vi "CRYReplace Analysis Curve Name.vi"(7 "Setup in":T1={"No.VI"=0, "Category"="", "StepName"="", "Seq setup flattened"="", "Comment"="", "Steps config."=[], "Jump config"=[], "Start"=0.0, "Increment"=0.0, "Name"="Pa", "Unit"="Pa", "Y data"=1, "Y prefix"="", "Y dB ref"=1.0, "Y unit"="", "Repeat State Array"=[]} {"Repeat State Array"."Start" format="%#_5g"; "Y dB ref" format="%.1f"; "Y data" items=["dB", "Lin"]; "Start" format="%#_5g"}, 8 "Hardware Setup In":string, 9 "Step Setup In":string, 10 "InsertSocket?":bool, 11 "Type In":string) -> (0 "New Custom Name( Channel case)":string[](array[string]), 1 "Signal Type":string, 2 "Curve Info Array Out":T2(array[cluster]), 3 "Inserted Names Out":string[](array[string]), 5 "New Custom Type( Channel case)":string[](array[string]))   [LabVIEW 2013]
uses:
  Typedef Control/CRYData Cluster Array.ctl
  Typedef Control/CRYData Cluster.ctl
  Typedef Control/CRYWaveform Cluster.ctl
  Typedef Control/CRYStep.ctl
  Typedef Control/CRYAnalysis CurveName Cluster.ctl
  Typedef Control/CRYUnit Info Out Cluster.ctl
panel:
  in  "Wave out":T3[](array[typedef]) {"Y dB ref" format="%.1f"; "Y axis" items=["Log", "Lin"]; "Y data" items=["dB", "Lin"]; "X data" items=["dB", "Lin"]}
  in  "Curve array":T4 {"Z data" items=["dB", "Lin"]; "X data" items=["dB", "Lin"]; "Y data" items=["dB", "Lin"]; "Z dB ref" format="%.1f"; "Z axis" items=["Log", "Lin"]; "X dB ref" format="%.1f"; "X axis" items=["Log", "Lin"]; "Y axis" items=["Log", "Lin"]; "Y dB ref" format="%.1f"; "Curve"."z" format="%.2f"; "Curve"."y" format="%.2f"; "Curve"."x" format="%.2f"}
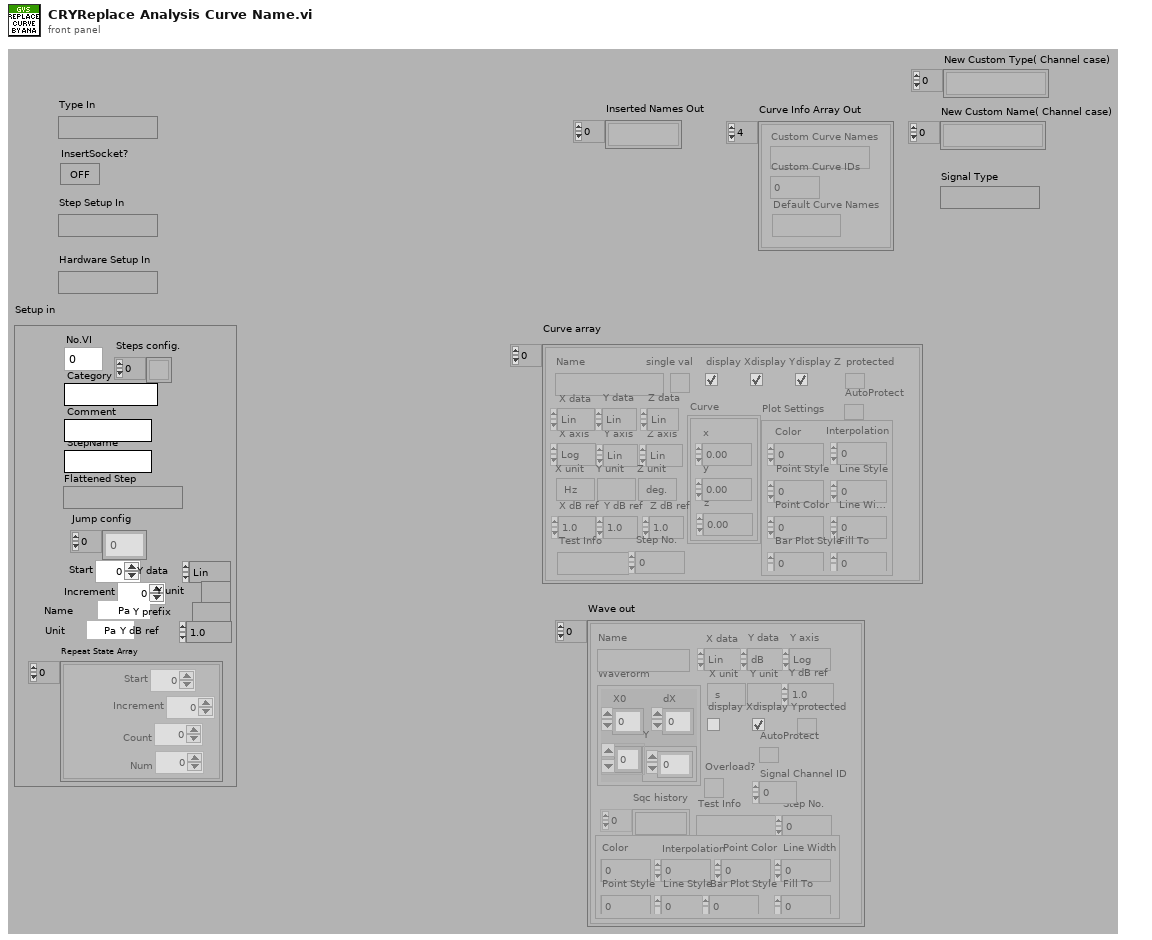
[diagram p1: front panel]
types:
  T1 = typedef "CRYStep.ctl" = cluster{"No.VI":i32, "Category":string, "StepName":string, "Seq setup flattened":string, "Comment":string, "Steps config.":bool[], "Jump config":i32[], "Start":dbl, "Increment":dbl, "Name":string, "Unit":string, "Y data":u16, "Y prefix":string, "Y dB ref":dbl, "Y unit":string, "Repeat State Array":cluster{"Start":dbl, "Increment":dbl, "Count":i32, "Num":i32}[]}
  T2 = cluster{"Custom Curve Names":string, "Custom Curve IDs":i32, "Default Curve Names":string}[]
  T3 = typedef "CRYWaveform Cluster.ctl" = cluster{"Waveform":cluster{"X0":dbl, "dX":dbl, "Y":sgl[]}, "X data":u16, "Y data":u16, "Y axis":u16, "X unit":string, "Y unit":string, "Y dB ref":dbl, "display Y":bool, "display X":bool, "Overload?":bool, "Test Info":string, "Step No.":i32, "Name":string, "protected":bool, "Sqc history":string[], "Signal Channel ID":i32, "Plot Settings":cluster{"Color":u32, "Interpolation":u8, "Point Style":u8, "Line Style":u8, "Point Color":u32, "Line Width":u8, "Bar Plot Style":u8, "Fill To":i16}, "AutoProtect":bool}
  T4 = typedef "CRYData Cluster Array.ctl" = T5[]
  T5 = typedef "CRYData Cluster.ctl" = cluster{"Name":string, "Curve":cluster{"x":dbl, "y":dbl, "z":dbl}[], "X data":u16, "Y data":u16, "Z data":u16, "X axis":u16, "Y axis":u16, "Z axis":u16, "X unit":string, "Y unit":string, "Z unit":string, "X dB ref":dbl, "Y dB ref":dbl, "Z dB ref":dbl, "single val":bool, "protected":bool, "display X":bool, "display Y":bool, "display Z":bool, "Test Info":string, "Step No.":i32, "Plot Settings":cluster{"Color":u32, "Interpolation":u8, "Point Style":u8, "Line Style":u8, "Point Color":u32, "Line Width":u8, "Bar Plot Style":u8, "Fill To":i16}, "AutoProtect":bool}
  T6 = cluster{"X unit":string, "X data":u16, "Y unit":string, "Y data":u16, "Z unit":string, "X data":u16, "dB ref":dbl}
  T7 = typedef "CRYUnit Info Out Cluster.ctl" = cluster{"X unit":string, "X data":u16, "Y unit":string, "Y data Time":u16, "Z unit":string, "X axis":u16, "X dB ref":dbl, "Y dB ref":dbl, "single/curve":bool}
  T8 = typedef "CRYAnalysis CurveName Cluster.ctl" = cluster{"Custom Curve Name":string, "Custom Curve ID":i32, "Default Curve Name":string}[]
  T9 = cluster{"display X":bool, "display Y":bool, "display Z":bool}[]
  T10 = cluster{"X unit":string, "X data":u16, "Y unit":string, "Y data":u16, "Z unit":string, "X data":u16, "dB ref":dbl}[]
  T11 = cluster{"Start":dbl, "Increment":dbl, "Count":i32, "Num":i32}[]
  T12 = typedef "CRYAnalysis Cluster.ctl" = cluster{"Name":string, "Harmonics":dbl[], " Algorithm":u16, "delay":dbl, "THD(%)":bool, "Rub&Buzz":bool, "Imp":bool, "Imp Ref resistor":dbl, "Y data":u16, "Y prefix":string, "Y unit":string, "Y dB ref":dbl, "Custom Curve Names":string[], "har list items":string[], "Envelope":bool, "use custom unit":bool, "autodelay ch":dbl, "impulse":bool, " start ms":dbl, " stop ms":dbl, "Scaling":i32, "Default Overlap ":bool, "Advanced View":bool, "Loose Particle":bool, "Use default":bool, "Auto-Correlation(Stimulus)":bool, "Auto-Correlation(Response)":bool, "Deconvolved Response":bool, "Mic Current":bool, "M List Vaiues":u16, "Type":u16, "Delay Method":u16, "Apply Correction Out":bool, "Apply Correction In":bool, "Harmonics @ meas.frq":bool, "THD Normalized(%)":bool, "Total Distortion":bool, "THD+Noise(%)":bool, "Rub&Buzz Norm'd(%)":bool, "Standard Error":bool, "Confidence Limits":bool, "Total Diff":bool, "Total Noise":bool, "Total DFD(%)":bool, "Total IMD(%)":bool, "Total IM":bool, "Total DFD+Noise(%)":bool, "Use Channel Name":bool, "Waveform In":string, "Waveform Out":string, "Method":u16, "Spectral Scaling":u16, "Appliied Unit":u16, "Length Unit":u16, "Applied Units":u16, "Sens Item":u16, "Tab":i32, "Distance Unit":u16, "discard cycles":dbl, "Weigting":string, "Averaging Time":dbl, "Max duration":dbl, "Min duration":dbl, "Attack Threshold":dbl, "Hysteresis Up":dbl, "Fmin(Hz)":dbl, "Fmax(Hz)":dbl, "Freq.Resolution":dbl, "Over-samples Res.":dbl, "Win Resolution":dbl, "distance":dbl, "samples":dbl, "Overlap":dbl, "Record Length":dbl, "No.of FFTs":dbl, "Hz":dbl, "record delay":dbl, " Std Err":dbl, "Response":bool, "Coherent Power*":bool, "Stimulus":bool, "Measurement Confidence":bool, "Auto Spectrum(Response)*":bool, "Auto Spectrum(Stimulus)*":bool, "Cross Spectrum*":bool, "functions":bool, "Frequency Response":bool, "Non-Coherent Power*":bool, "Coherence (%)":bool, "Non-Coherence (%)":bool, "Signal-Noise Ratio (dB)":bool, "Non-Coherenct Distirtion*":bool, "Result Waveforms":bool, "Coupling":bool, "Averaging":u16, "Harmonics":i32, "Custom Curve Names":i32, "unLabel":string, "Custom Curve Names":string, "Unit":string, "Total IMD + Noise(%) ":bool, "ResponseMe":u16, "Intermod":dbl[], "Diff\n":dbl[], "Cross-Correlation":bool, "IM list items":string[], "Diff list items":string[], "TSR Window Type":string, "Help":string, "Custom Curve IDs":i32[], "Default Curve Names":string[], "Loose Particle waveform":bool, "Perceptual Rub&Buzz":bool, "Imp Auto Mode":u16, "Mic Auto Mode":u16, "Mic Ref resistor":dbl, "Curve Resolution":u16, "Curve Resolution Hz":dbl, "Polarity":bool}
  T13 = typedef "CRYStimulus Test Infor Cluster.ctl" = cluster{"Stimulus Type":string, "Signal Type":string, "In/Out":bool, "FAPS":cluster{"freq":dbl, "ampl":dbl, "cycles":dbl, "samples":i32}[], "Sampling Rate":dbl, "Samples":i32, "Analysis Param":string, "Resolution":u16, "Steps":u32, "Analysis Value":dbl[], "Diff Freq":dbl, "FStart":dbl, "FStop":dbl, "Calibration Param":string, "Anti Alias":dbl, "Level Out1":dbl, "Level Out2":dbl, "EQ":bool}
  T14 = typedef "CRYCalibration 2DCluster.ctl" = cluster{"Calibration":T15, "Corr Curve":T5, "EQ Curve":T5, "Sens Curve":T5}
  T15 = typedef "CRYCalibration Cluster.ctl" = cluster{"Calibration Step Name":string, "Device":string, "Correction Curve Name":string, "Equalization Curve Name":string, "Sensitivity Curve Name":string, "Corr Folder and File":string, "EQ Folder and File":string, "Sens Folder and File":string, "Corr Step size":u16, "EQ Step size":u16, "Input":bool, "Last Cal Date (sec)":timestamp, "Cha Name":string, "Corr Curve Found":bool, "EQ Curve Found":bool, "Sens Curve Found":bool, "Signal Type":string, "Calibrated Device":string, "Hz":u32}
  T16 = cluster{bool, "Check Option":string, "use custom unit":bool, "Custom Curve Names":string[], "Custom Curve IDs":i32[], "Default Curve Names":string[], "Use default":bool}
  T17 = cluster{"Y unit":string, "Y dB ref":dbl, "Y unit":string, "Y dB ref":dbl, "Y unit":string, "Y dB ref":dbl, "Y data":u16, u16}
  T18 = cluster{"X unit":string, "X data":u16, "Y unit":string, "X data":u16, "Y unit":string, "X data":u16, "dB ref In":dbl}[]
  T19 = cluster{"X unit":string, "X data":u16, "Y unit":string, "Y data Time":u16, "Z unit":string, "X data":u16, "dB ref":dbl}[]
  T20 = typedef "CRYWaveform Cluster Array.ctl" = T3[]
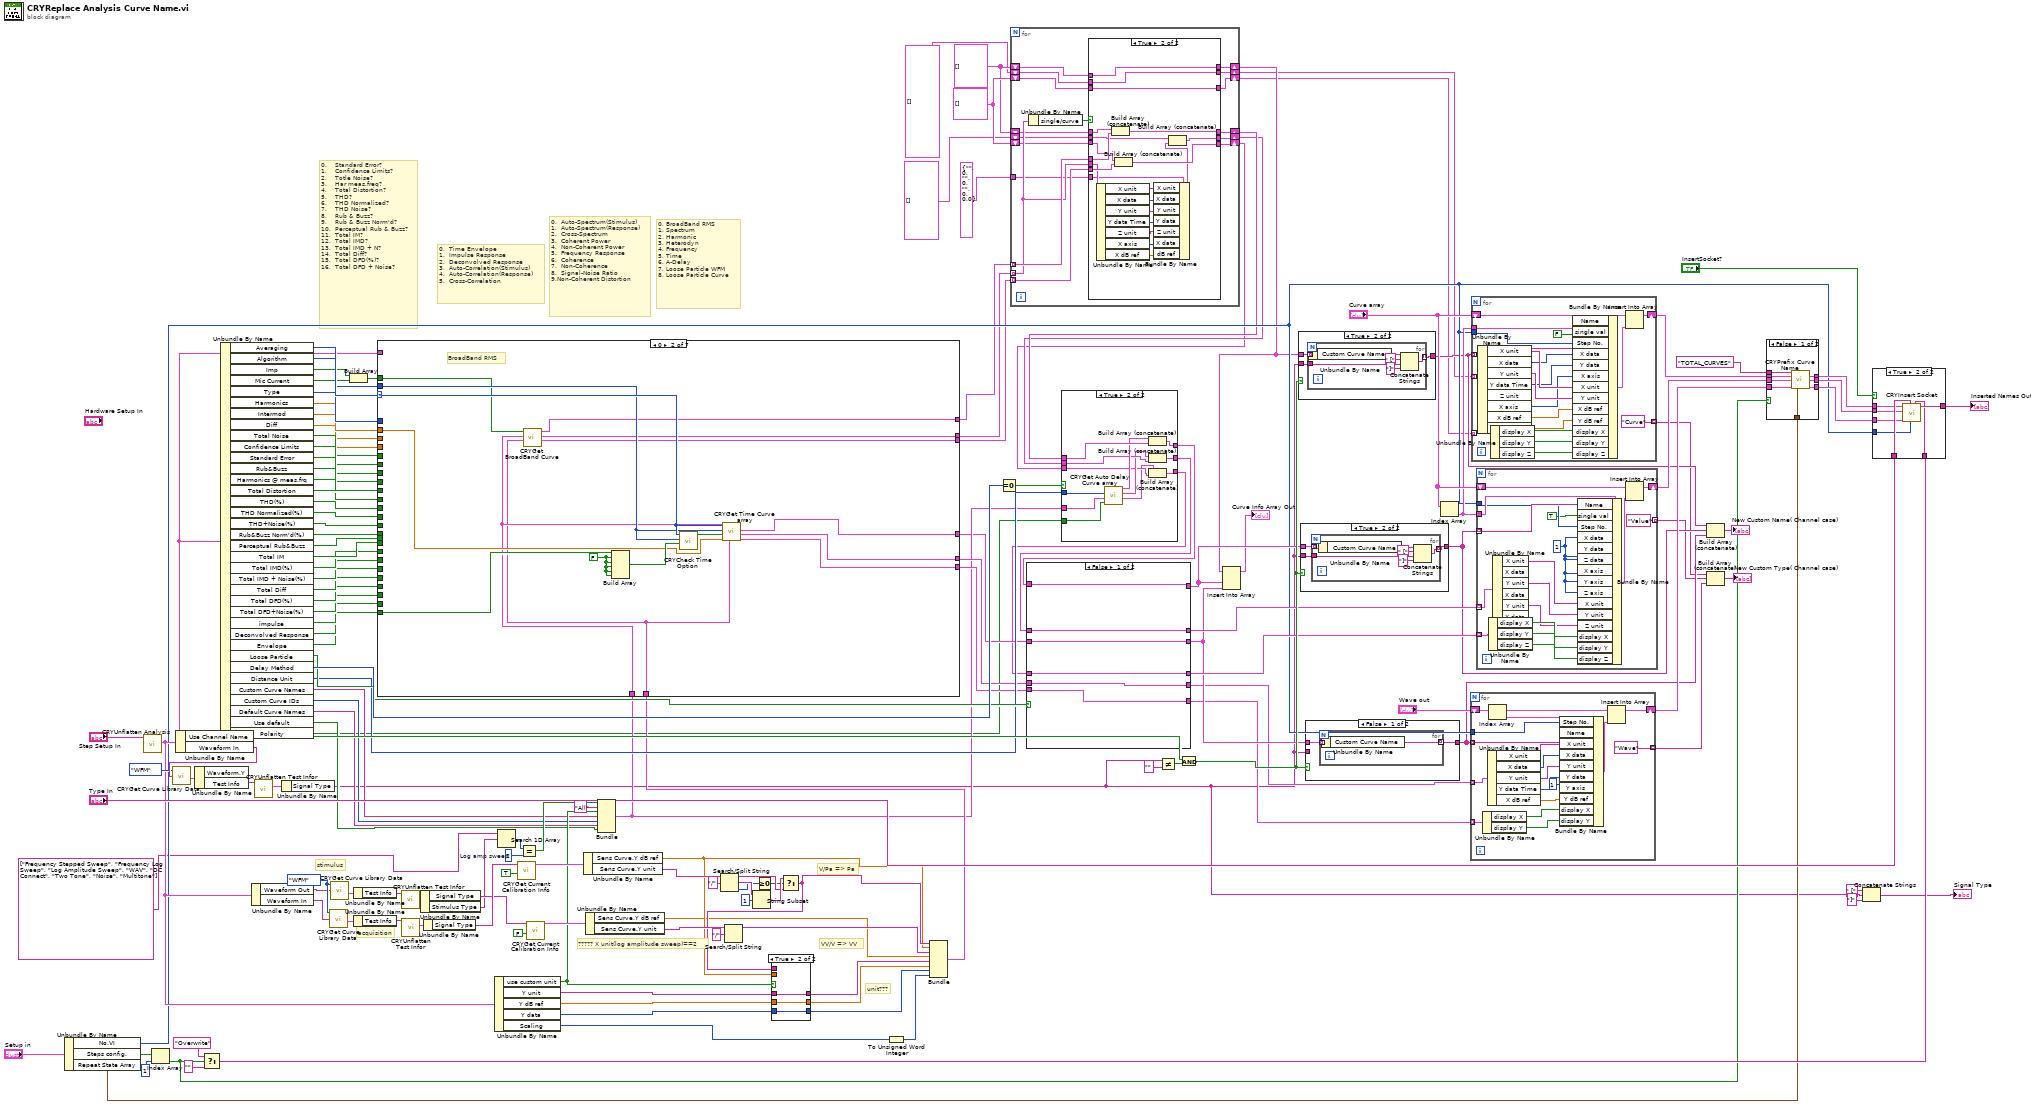
[diagram p0: block diagram]
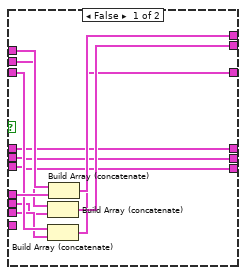
[diagram p2: hidden frame]
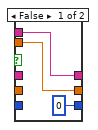
[diagram p5: hidden frame]
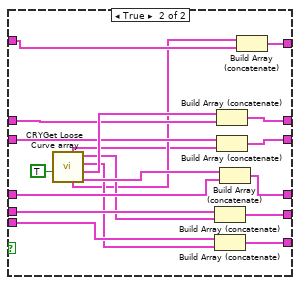
[diagram p7: hidden frame]
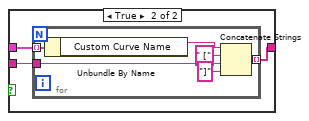
[diagram p8: hidden frame]
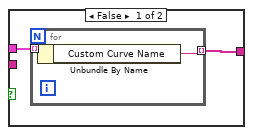
[diagram p9: hidden frame]
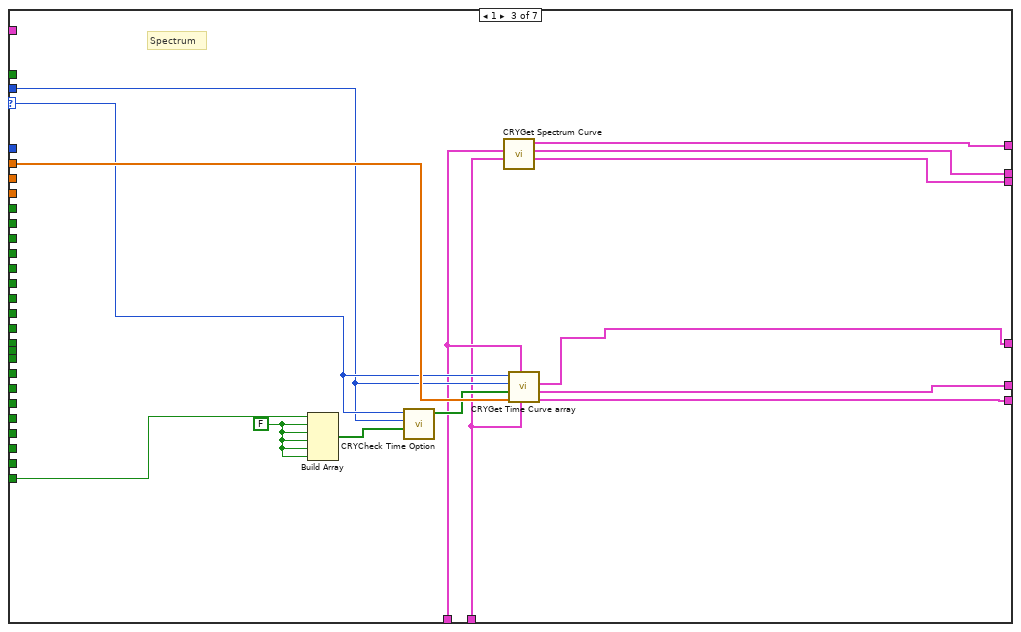
[diagram p11: hidden frame]
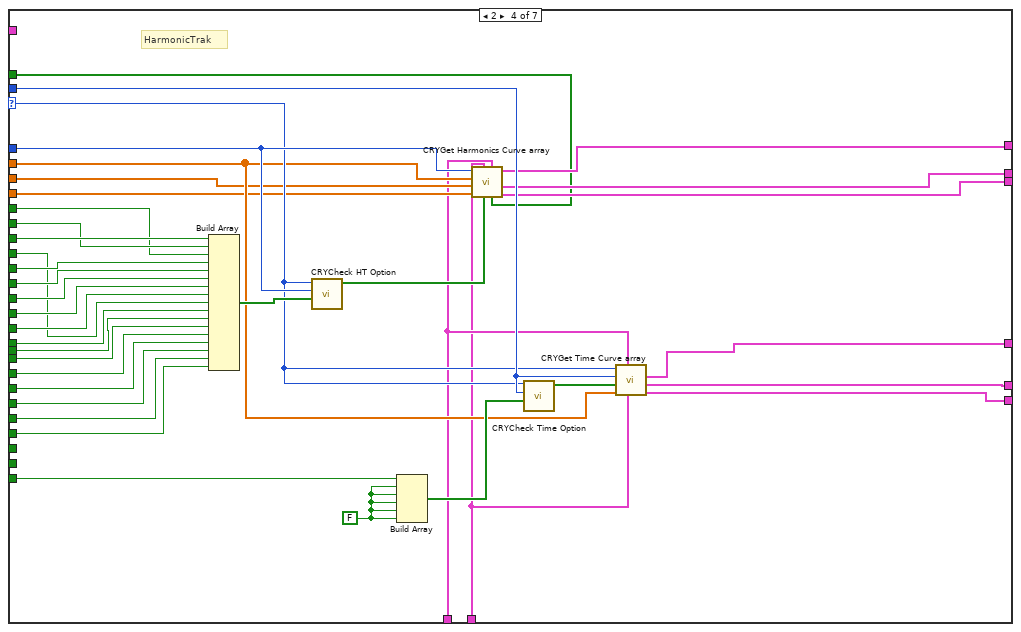
[diagram p12: hidden frame]
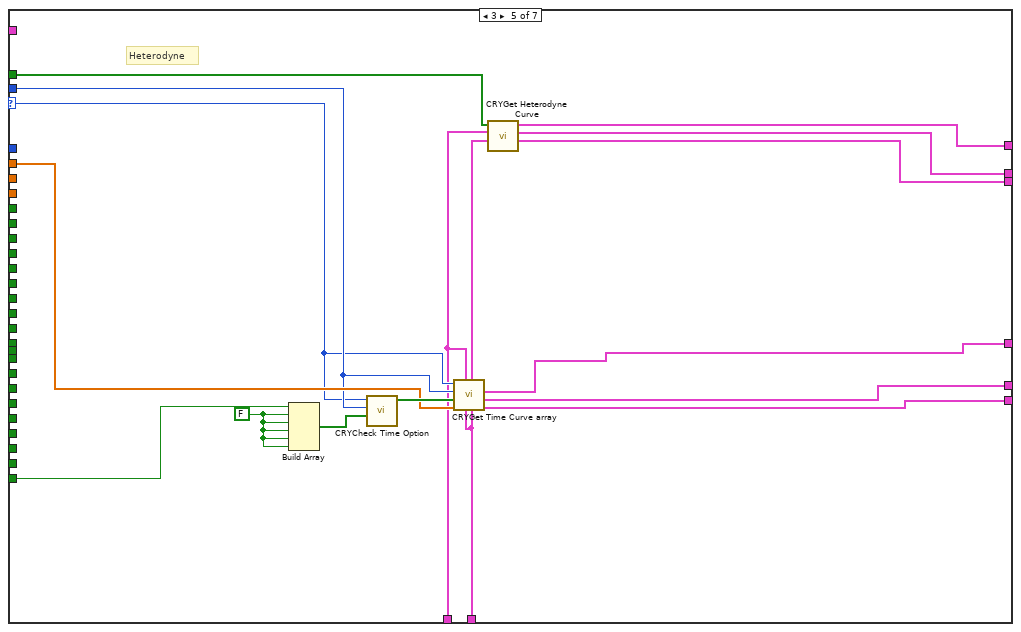
[diagram p13: hidden frame]
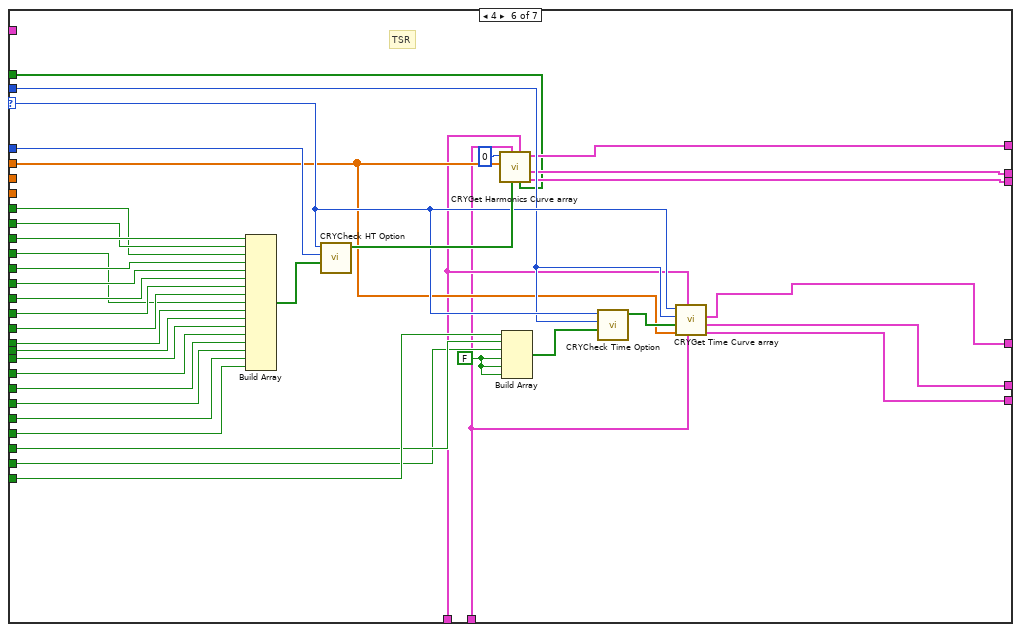
[diagram p14: hidden frame]
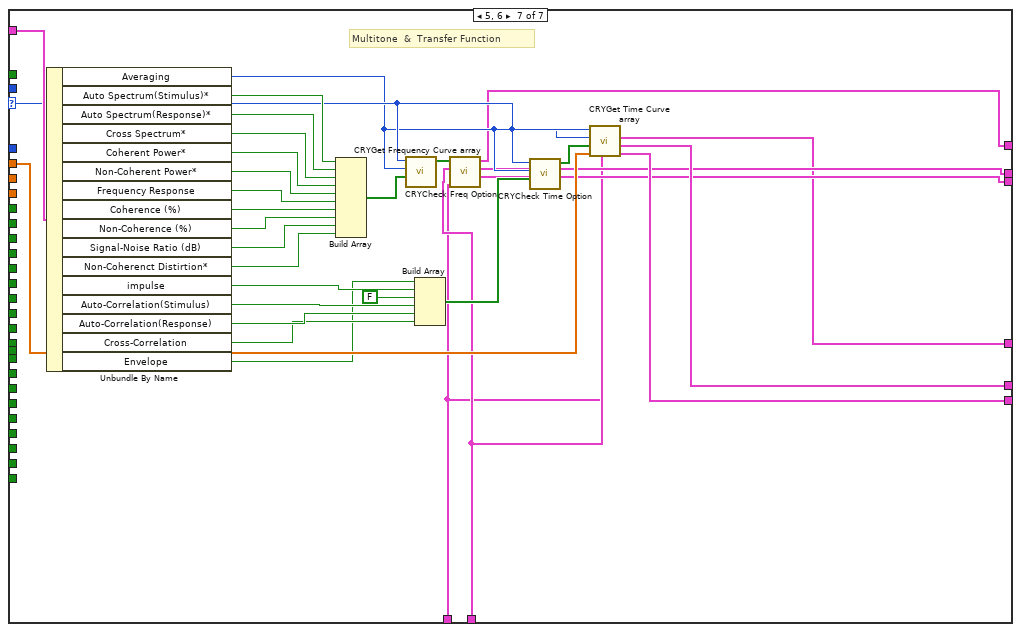
[diagram p15: hidden frame]
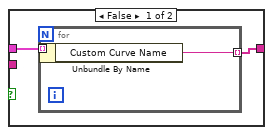
[diagram p16: hidden frame]
diagram:
  w13 = T8 [] ("Curve Info Array Out")
  w15 = T9 []
  w72 = 2  # Log amp sweep
  w82 = enum16{"Curves", "Values", "Results", "WFM"}."WFM" ("Type")
  # "0, BroadBand RMS\n1, Spectrum\n2, Harmonic\n3, Heterodyn\n4, Frequency\n5, Time\n6, A-Delay\n7, Loose Particle WFM\n8, Loose Particle Curve"
  # "acquisition"
  # "stimulus"
  # "unit???"
  # "V/Pa => Pa"
  # "VV/V => VV"
  # "????? X unit(log amplitude sweep)==2"
  # "0,  Auto-Spectrum(Stimulus)\n1,  Auto-Spectrum(Response)\n2,  Cross-Spectrum\n3,  Coherent Power\n4,  Non-Coherent Power\n5,  Frequency Response\n6,  Coherence\n7,  Non-Coherence\n8,  Signal-Noise Ratio\n9,Non-Coherent Distortion"
  # "0,    Standard Error?\n1,    Confidence Limits?\n2,    Totle Noise?\n3,    Har meas.freq?\n4,    Total Distortion?\n5,    THD?\n6,    THD Normalized?\n7,    THD Noise?\n8,    Rub & Buzz?\n9,    Rub & Buzz Norm'd?\n10,  Perceptual Rub & Buzz?\n11,  Total IM?\n12,  Total IMD?\n13,  Total IMD + N?\n14,  Total Diff?\n15,  Total DFD(%)?\n16,  Total DFD + Noise?"
  # "0,  Time Envelope\n1,  Impulse Response\n2,  Deconvolved Response\n3,  Auto-Correlation(Stimulus)\n4,  Auto-Correlation(Response)\n5,  Cross-Correlation"
  n1 = Unbundle By Name("Setup in") -> ("No.VI"=w37:i32, "Steps config."=w47:bool[], "Repeat State Array"=w39:T11)
  n2 = call "CRYUnflatten Analysis.vi"("Unflatten Analysis"="Step Setup In") -> ("Analysis"=w75:T12)  [unwired: 8 in, 2 out]
  n3 = Index Array(array=w47, index=1) -> (element=w38:bool)
  n4 = Unbundle By Name(w75) -> ("Use Channel Name"=w124:bool, "Waveform In"=w155:string)
  n5 = call "CRYGet Curve Library Data.vi"("Type"=enum16{"Curves", "Values", "Results", "WFM"}."WFM", "Data Name"=w155) -> ("Wave"=w153:T3)  [unwired: 4 out]
  n6 = Unbundle By Name(w153) -> ("Test Info"=w152:string)  [unwired: 1 out]
  n7 = Select(t="Overwrite" ("Y unit"), s=w38, f="") -> (s? t:f=w49:string)
  n8 = Unbundle By Name(w75) -> ("Averaging"=w120:u16, "Algorithm"=w150:u16, "Imp"=w22:bool, "Mic Current"=w21:bool, "Type"=w149:u16, "Harmonics"=w148:dbl[], "Intermod"=w137:dbl[], "Diff"=w133:dbl[], "Total Noise"=w138:bool, "Confidence Limits"=w139:bool, "Standard Error"=w140:bool, "Rub&Buzz"=w141:bool, "Harmonics @ meas.frq"=w147:bool, "Total Distortion"=w146:bool, "THD(%)"=w145:bool, "THD Normalized(%)"=w144:bool, "THD+Noise(%)"=w143:bool, "Rub&Buzz Norm'd(%)"=w142:bool, "Perceptual Rub&Buzz"=w35:bool, "Total IM"=w136:bool, "Total IMD(%)"=w135:bool, "Total IMD + Noise(%)"=w134:bool, "Total Diff"=w132:bool, "Total DFD(%)"=w131:bool, "Total DFD+Noise(%)"=w130:bool, "impulse"=w129:bool, "Deconvolved Response"=w128:bool, "Envelope"=w121:bool, "Loose Particle"=w116:bool, "Delay Method"=w127:u16, "Distance Unit"=w114:u16, "Custom Curve Names"=w60:string[], "Custom Curve IDs"=w59:i32[], "Default Curve Names"=w58:string[], "Use default"=w57:bool, "Polarity"=w19:bool)
  n9 = Unbundle By Name(w75) -> ("Waveform Out"=w80:string, "Waveform In"=w81:string)
  n10 = call "CRYUnflatten Test Infor.vi"("Falattend test infor"=w152) -> ("unflattened test infor data"=w151:T13)  [unwired: 9 out]
  n11 = Unbundle By Name(w151) -> ("Signal Type"=w28:string)
  n12 = call "CRYGet Curve Library Data.vi"("Type"=w82, "Data Name"=w81) -> ("Wave"=w84:T3)  [unwired: 4 out]
  n13 = call "CRYGet Curve Library Data.vi"("Type"=w82, "Data Name"=w80) -> ("Wave"=w83:T3)  [unwired: 4 out]
  n14 = Build Array(w22, w21) -> (w20:bool[])
  n15 = Unbundle By Name(w83) -> ("Test Info"=w76:string)
  n16 = Unbundle By Name(w84) -> ("Test Info"=w78:string)
  n17 = call "CRYUnflatten Test Infor.vi"("Falattend test infor"=w76) -> ("unflattened test infor data"=w79:T13)  [unwired: 9 out]
  n18 = call "CRYUnflatten Test Infor.vi"("Falattend test infor"=w78) -> ("unflattened test infor data"=w77:T13)  [unwired: 9 out]
  n19 = Unbundle By Name(w79) -> ("Signal Type"=w73:string, "Stimulus Type"=w70:string)
  n20 = Unbundle By Name(w77) -> ("Signal Type"=w74:string)
  n21 = Unbundle By Name(w75) -> ("use custom unit"=w61:bool, "Y unit"=w95:string, "Y dB ref"=w96:dbl, "Y data"=w94:u16, "Scaling"=w93:i32)
  n22 = Search 1D Array(1D array=string[] ["Frequency Stepped Sweep", "Frequency Log Sweep", "Log Amplitude Sweep", "WAV", "DC Connect", "Two Tone", "Noise", "Multitone"] ("Strings []"), element=w70) -> (index of element=w71:i32)  [unwired: 1 out]
  n23 = call "CRYGet Current Calibration Info.vi"("Is Input?"=TRUE, "Signal Type Name"=w74) -> ("Calibration All Cluster"=w106:T14)  [unwired: 9 out]
  n24 = Equal?(x=w71, y=w72) -> (x = y?=w69:bool)
  n25 = call "CRYGet Current Calibration Info.vi"("Is Input?"=FALSE, "Signal Type Name"=w73) -> ("Calibration All Cluster"=w109:T14)  [unwired: 9 out]
  n26 = Unbundle By Name(w106) -> ("Sens Curve.Y dB ref"=w90:dbl, "Sens Curve.Y unit"=w97:string)
  n27 = Unbundle By Name(w109) -> ("Sens Curve.Y dB ref"=w88:dbl, "Sens Curve.Y unit"=w105:string)
  n28 = Bundle(w69, "Check Option"="All", "use custom unit"=w61, "Custom Curve Names"=w60, "Custom Curve IDs"=w59, "Default Curve Names"=w58, "Use default"=w57) -> (w56:T16)  [unwired: 1 in]
  n29 = Search/Split String(string=w97, search string/char (-)="/" ("search char (-)")) -> (substring before match=w101:string, match + rest of string=w103:string, offset of match=w99:i32)  [unwired: 1 out]
  n30 = Search/Split String(string=w105, search string/char (-)="/" ("search char (-)")) -> (substring before match=w89:string)  [unwired: 3 out]
  n31 = String Subset(string=w103, offset (0)=1) -> (substring=w104:string)  [unwired: 1 in]
  n32 = Greater Or Equal To 0?(x=w99) -> (x >= 0?=w100:bool)
  n33 = Select(t=w104, s=w100, f=w101) -> (s? t:f=w91:string)
  n34 = case shown="True" w61 {
    tunnel: w96 -> [_ w161]
    tunnel: w95 -> [_ w162]
    tunnel: [w158 w162] -> w87
    tunnel: w90 -> [w159 _]
    tunnel: w91 -> [w158 _]
    tunnel: [w159 w161] -> w86
    tunnel: w94 -> [_ w160]
    tunnel: [u16 0 ("Y data") w160] -> w85
    frame False {
    }
    frame True {
    }
  }
  n35 = To Unsigned Word Integer(number=w93) -> (unsigned 16bit integer=w92:u16)
  n36 = Bundle("Y unit"=w91, "Y dB ref"=w90, "Y unit"=w89, "Y dB ref"=w88, "Y unit"=w87, "Y dB ref"=w86, "Y data"=w85, w92) -> (w67:T17)  [unwired: 1 in]
  n37 = case shown="0" w150 {
    selector: w150 -> [_ w173 w188 w207 w241 w260 w299]
    tunnel: w149 -> [_ _ _ w214 _ w268 _]
    tunnel: w148 -> [_ w174 w190 w206 w243 w258 w296]
    tunnel: w147 -> [_ _ _ w231 _ w282 _]
    tunnel: w146 -> [_ _ _ w230 _ w281 _]
    tunnel: w145 -> [_ _ _ w229 _ w280 _]
    tunnel: w144 -> [_ _ _ w228 _ w279 _]
    tunnel: w143 -> [_ _ _ w227 _ w278 _]
    tunnel: w142 -> [_ _ _ w226 _ w276 _]
    tunnel: w141 -> [_ _ _ w225 _ w277 _]
    tunnel: w140 -> [_ _ _ w224 _ w285 _]
    tunnel: w139 -> [_ _ _ w223 _ w284 _]
    tunnel: w138 -> [_ _ _ w216 _ w283 _]
    tunnel: w137 -> [_ _ _ w205 _ _ _]
    tunnel: w136 -> [_ _ _ w222 _ w275 _]
    tunnel: w135 -> [_ _ _ w221 _ w274 _]
    tunnel: w134 -> [_ _ _ w220 _ w273 _]
    tunnel: w133 -> [_ _ _ w204 _ _ _]
    tunnel: w132 -> [_ _ _ w219 _ w272 _]
    tunnel: w131 -> [_ _ _ w218 _ w271 _]
    tunnel: w130 -> [_ _ _ w217 _ w270 _]
    tunnel: w129 -> [_ _ _ _ _ w265 _]
    tunnel: w128 -> [_ _ _ _ _ w264 _]
    tunnel: w75 -> [_ _ _ _ _ _ w318]
    tunnel: [_ w166 w181 w198 w235 w252 w288] -> w18
    tunnel: [_ w167 w182 w199 w236 w253 w289] -> w55
    tunnel: w121 -> [_ w177 w192 w211 w247 w266 _]
    tunnel: w120 -> [_ w172 w187 w208 w242 w259 _]
    tunnel: w56 -> [_ w165 w180 w197 w234 w251 w287]
    tunnel: w67 -> [_ w164 w179 w196 w233 w250 w290]
    tunnel: [_ w171 w186 w201 w238 w255 w294] -> w65
    tunnel: [_ w170 w185 w200 w237 w254 w293] -> w64
    tunnel: [_ w169 w184 w203 w240 w257 w291] -> w17
    tunnel: [_ w168 w183 w202 w239 w256 w292] -> w16
    tunnel: w35 -> [_ _ _ w195 _ w249 _]
    tunnel: w20 -> [_ w163 _ w194 w232 w248 _]
    frame Default {
    }
    frame 0 {
      w178 = FALSE ("element")
      # "BroadBand RMS"
      n38 = call "CRYGet BroadBand Curve.vi"("Unit Info In"=w164, "Additive Info"=w165, "Impedance and Mic Current In"=w163) -> ("Display Array"=w168:T9, "Unit Info Out"=w169:T7[], "Curve Info Array Out"=w166:T8)  [unwired: 6 in]
      n39 = Build Array(w177, w178, w178, w178, w178, w178) -> (w176:bool[])
      n40 = call "CRYCheck Time Option.vi"("Option Array In"=w176, "Averaging"=w172, "Algorithm"=w173) -> ("Option Array Out"=w175:bool[])  [unwired: 8 in]
      n41 = call "CRYGet Time Curve array.vi"("Unit Info In"=w164, "Additive Info"=w165, "Harmonics array"=w174, "Option Array In"=w175, "Averaging"=w172, "Algorithm"=w173) -> ("Display Array"=w170:T9, "Unit Info Out"=w171:T7[], "Curve Info Array Out"=w167:T8)  [unwired: 3 in]
    }
    frame 1 {
      w193 = FALSE ("element")
      # "Spectrum"
      n42 = Build Array(w192, w193, w193, w193, w193, w193) -> (w191:bool[])
      n43 = call "CRYCheck Time Option.vi"("Option Array In"=w191, "Averaging"=w187, "Algorithm"=w188) -> ("Option Array Out"=w189:bool[])  [unwired: 8 in]
      n44 = call "CRYGet Spectrum Curve.vi"("Unit Info In"=w179, "Additive Info"=w180) -> ("Display Array"=w183:T9, "Unit Info Out"=w184:T7[], "Curve Info Array Out"=w181:T8)  [unwired: 7 in]
      n45 = call "CRYGet Time Curve array.vi"("Unit Info In"=w179, "Additive Info"=w180, "Harmonics array"=w190, "Option Array In"=w189, "Averaging"=w187, "Algorithm"=w188) -> ("Display Array"=w185:T9, "Unit Info Out"=w186:T7[], "Curve Info Array Out"=w182:T8)  [unwired: 3 in]
    }
    frame 2 {
      w212 = FALSE ("element")
      # "HarmonicTrak"
      n46 = Build Array(w224, w223, w216, w231, w230, w229, w228, w227, w225, w226, w195, w222, w221, w220, w219, w218, w217) -> (w215:bool[])
      n47 = call "CRYCheck HT Option.vi"("Option Array In"=w215, "Type"=w214, "Algorithm"=w207) -> ("Option Array Out"=w213:bool[])  [unwired: 8 in]
      n48 = Build Array(w211, w212, w212, w212, w212, w212) -> (w210:bool[])
      n49 = call "CRYGet Harmonics Curve array.vi"("Impedance and Mic Current In"=w194, "Additive Info"=w197, "Option Array In"=w213, "Unit Info"=w196, "Diff array"=w204, "IM array"=w205, "Harmonics array"=w206, "Type"=w214) -> ("Display Array"=w202:T9, "Unit Info Out"=w203:T7[], "Curve Info Array Out"=w198:T8)  [unwired: 1 out]
      n50 = call "CRYCheck Time Option.vi"("Option Array In"=w210, "Averaging"=w208, "Algorithm"=w207) -> ("Option Array Out"=w209:bool[])  [unwired: 8 in]
      n51 = call "CRYGet Time Curve array.vi"("Unit Info In"=w196, "Additive Info"=w197, "Harmonics array"=w206, "Option Array In"=w209, "Averaging"=w208, "Algorithm"=w207) -> ("Display Array"=w200:T9, "Unit Info Out"=w201:T7[], "Curve Info Array Out"=w199:T8)  [unwired: 3 in]
    }
    frame 3 {
      w246 = FALSE ("element")
      # "Heterodyne"
      n52 = Build Array(w247, w246, w246, w246, w246, w246) -> (w245:bool[])
      n53 = call "CRYCheck Time Option.vi"("Option Array In"=w245, "Averaging"=w242, "Algorithm"=w241) -> ("Option Array Out"=w244:bool[])  [unwired: 8 in]
      n54 = call "CRYGet Time Curve array.vi"("Unit Info In"=w233, "Additive Info"=w234, "Harmonics array"=w243, "Option Array In"=w244, "Averaging"=w242, "Algorithm"=w241) -> ("Display Array"=w237:T9, "Unit Info Out"=w238:T7[], "Curve Info Array Out"=w236:T8)  [unwired: 3 in]
      n55 = call "CRYGet Heterodyne Curve.vi"("Unit Info In"=w233, "Additive Info"=w234, "Impedance and Mic Current In"=w232) -> ("Display Array"=w239:T9, "Unit Info Out"=w240:T7[], "Curve Info Array Out"=w235:T8)  [unwired: 6 in]
    }
    frame 4 {
      w263 = FALSE ("element")
      # "TSR"
      n56 = Build Array(w285, w284, w283, w282, w281, w280, w279, w278, w277, w276, w249, w275, w274, w273, w272, w271, w270) -> (w269:bool[])
      n57 = call "CRYCheck HT Option.vi"("Option Array In"=w269, "Type"=w268, "Algorithm"=w260) -> ("Option Array Out"=w267:bool[])  [unwired: 8 in]
      n58 = call "CRYGet Harmonics Curve array.vi"("Impedance and Mic Current In"=w248, "Additive Info"=w251, "Option Array In"=w267, "Unit Info"=w250, "Harmonics array"=w258, "Type"=u16 0) -> ("Display Array"=w256:T9, "Unit Info Out"=w257:T7[], "Curve Info Array Out"=w252:T8)  [unwired: 2 in, 1 out]
      n59 = Build Array(w266, w265, w264, w263, w263, w263) -> (w262:bool[])
      n60 = call "CRYCheck Time Option.vi"("Option Array In"=w262, "Averaging"=w259, "Algorithm"=w260) -> ("Option Array Out"=w261:bool[])  [unwired: 8 in]
      n61 = call "CRYGet Time Curve array.vi"("Unit Info In"=w250, "Additive Info"=w251, "Harmonics array"=w258, "Option Array In"=w261, "Averaging"=w259, "Algorithm"=w260) -> ("Display Array"=w254:T9, "Unit Info Out"=w255:T7[], "Curve Info Array Out"=w253:T8)  [unwired: 3 in]
    }
    frame 5, 6 {
      # "Multitone  &  Transfer Function"
      n62 = Unbundle By Name(w318) -> ("Averaging"=w298:u16, "Auto Spectrum(Stimulus)*"=w317:bool, "Auto Spectrum(Response)*"=w316:bool, "Cross Spectrum*"=w315:bool, "Coherent Power*"=w314:bool, "Non-Coherent Power*"=w313:bool, "Frequency Response"=w312:bool, "Coherence (%)"=w311:bool, "Non-Coherence (%)"=w310:bool, "Signal-Noise Ratio (dB)"=w309:bool, "Non-Coherenct Distirtion*"=w308:bool, "impulse"=w305:bool, "Auto-Correlation(Stimulus)"=w303:bool, "Auto-Correlation(Response)"=w302:bool, "Cross-Correlation"=w301:bool, "Envelope"=w295:bool)
      n63 = Build Array(w317, w316, w315, w314, w313, w312, w311, w310, w309, w308) -> (w307:bool[])
      n64 = call "CRYCheck Freq Option.vi"("Option Array In"=w307, "Averaging"=w298, "Algorithm"=w299) -> ("Option Array Out"=w306:bool[])  [unwired: 8 in]
      n65 = Build Array(w295, w305, FALSE ("element"), w303, w302, w301) -> (w300:bool[])
      n66 = call "CRYGet Frequency Curve array.vi"("Additive Info"=w287, "Unit Info In"=w290, "Option Array In"=w306) -> ("Display Array"=w292:T9, "Unit Info Out"=w291:T7[], "Curve Info Array Out"=w288:T8)  [unwired: 6 in]
      n67 = call "CRYCheck Time Option.vi"("Option Array In"=w300, "Averaging"=w298, "Algorithm"=w299) -> ("Option Array Out"=w297:bool[])  [unwired: 8 in]
      n68 = call "CRYGet Time Curve array.vi"("Unit Info In"=w290, "Additive Info"=w287, "Harmonics array"=w296, "Option Array In"=w297, "Averaging"=w298, "Algorithm"=w299) -> ("Display Array"=w293:T9, "Unit Info Out"=w294:T7[], "Curve Info Array Out"=w289:T8)  [unwired: 3 in]
    }
  }
  n69 = Equal To 0?(x=w127) -> (x = 0?=w115:bool)
  n70 = for {
    tunnel: w18 -> [w333] mode=indexing
    tunnel: w17 -> [w332] mode=indexing
    tunnel: w16 -> [w331] mode=indexing
    shift-right: [w325] -> w10
    shift-left: w13 -> [w334]
    shift-right: [w324] -> w9
    shift-left: T7[] [] -> [w327]
    shift-right: [w323] -> w8
    shift-left: w15 -> [w326]
    shift-right: [w322] -> w7
    shift-left: w13 -> [w330]
    shift-right: [w321] -> w6
    shift-left: T10 [] -> [w329]
    shift-right: [w320] -> w5
    shift-left: w15 -> [w328]
    tunnel: T6 {"X unit"="", "X data"=0, "Y unit"="", "Y data"=0, "Z unit"="", "X data"=0, "dB ref"=0.0} ("Value Unit Info Out") -> [w319]
    n71 = Unbundle By Name(w332) -> ("single/curve"=w335:bool)
    n72 = case shown="True" w335 {
      tunnel: w334 -> [w347 w368]
      tunnel: w333 -> [w346 w364]
      tunnel: w332 -> [w339 w357]
      tunnel: w331 -> [w340 w361]
      tunnel: w330 -> [w338 w365]
      tunnel: w329 -> [w337 w359]
      tunnel: w328 -> [w336 w362]
      tunnel: w327 -> [w344 w367]
      tunnel: w326 -> [w342 w366]
      tunnel: [w345 w368] -> w325
      tunnel: [w343 w367] -> w324
      tunnel: [w341 w366] -> w323
      tunnel: [w338 w363] -> w322
      tunnel: [w337 w358] -> w321
      tunnel: [w336 w360] -> w320
      tunnel: w319 -> [_ w348]
      frame False {
        n73 = Build Array (concatenate)(w344, w339) -> (w343:T7[])
        n74 = Build Array (concatenate)(w342, w340) -> (w341:T9)
        n75 = Build Array (concatenate)(w347, w346) -> (w345:T8)
      }
      frame True {
        n76 = Unbundle By Name(w357) -> ("X unit"=w356:string, "X data"=w355:u16, "Y unit"=w354:string, "Y data Time"=w353:u16, "Z unit"=w352:string, "X axis"=w351:u16, "X dB ref"=w350:dbl)
        n77 = Build Array (concatenate)(w365, w364) -> (w363:T8)
        n78 = Build Array (concatenate)(w362, w361) -> (w360:T9)
        n79 = Bundle By Name(cluster=w348, "X unit"=w356, "X data"=w355, "Y unit"=w354, "Y data"=w353, "Z unit"=w352, "X data"=w351, "dB ref"=w350) -> (w349:T6)
        n80 = Build Array (concatenate)(w359, w349) -> (w358:T10)
      }
    }
  }
  n81 = case shown="True" w115 {
    tunnel: w114 -> [_ w383]
    tunnel: w56 -> [_ w382]
    tunnel: w19 -> [_ w381]
    tunnel: w7 -> [w371 w380]
    tunnel: w6 -> [w370 w375]
    tunnel: w5 -> [w369 w373]
    tunnel: [w371 w379] -> w4
    tunnel: [w370 w378] -> w3
    tunnel: [w369 w377] -> w2
    frame False {
    }
    frame True {
      n82 = call "CRYGet Auto Delay Curve array.vi"("Polarity"=w381, "Additive Info"=w382, "Distance Unit"=w383) -> ("Value Display Array"=w372:T9, "Value Unit Info Out"=w374:T18, "Curve Info Array Out"=w376:T8)  [unwired: 6 in]
      n83 = Build Array (concatenate)(w376, w380) -> (w379:T8)
      n84 = Build Array (concatenate)(w374, w375) -> (w378:T10)
      n85 = Build Array (concatenate)(w372, w373) -> (w377:T9)
    }
  }
  n86 = case shown="False" w116 {
    tunnel: w55 -> [w385 w396]
    tunnel: [w385 w395] -> w66
    tunnel: w4 -> [w384 w393]
    tunnel: w3 -> [w389 w406]
    tunnel: w2 -> [w388 w404]
    tunnel: [w389 w394] -> w112
    tunnel: [w388 w408] -> w113
    tunnel: w65 -> [w387 w402]
    tunnel: w64 -> [w386 w400]
    tunnel: [w387 w398] -> w63
    tunnel: [w386 w397] -> w62
    tunnel: [w384 w392] -> w54
    frame False {
    }
    frame True {
      n87 = call "CRYGet Loose Curve array.vi"("Loose Particle Waveform"=TRUE) -> ("Value Display Array"=w405:T9, "Value Unit Info Out"=w407:T19, "WMF Display Array"=w399:T9, "WFM Unit Info Out"=w401:T7[], "Curve Info Array Out"=w391:T8, "WFM Info Array Out"=w390:T8)  [unwired: 5 in]
      n88 = Build Array (concatenate)(w402, w401) -> (w398:T7[])
      n89 = Build Array (concatenate)(w400, w399) -> (w397:T9)
      n90 = Build Array (concatenate)(w407, w406) -> (w394:T10)
      n91 = Build Array (concatenate)(w396, w390) -> (w395:T8)
      n92 = Build Array (concatenate)(w405, w404) -> (w408:T9)
      n93 = Build Array (concatenate)(w391, w393) -> (w392:T8)
    }
  }
  n94 = Not Equal?(x=w28, y="") -> (x != y?=w125:bool)
  n95 = And(x=w124, y=w125) -> (x .and. y?=w117:bool)
  n96 = Insert Into Array(array=w10, new element #1=w54, new element #2=w66) -> (→"Curve Info Array Out":T8)  [unwired: 1 in]
  n97 = case shown="True" w117 {
    tunnel: w10 -> [w410 w415]
    tunnel: [w409 w414] -> w34
    tunnel: w28 -> [_ w413]
    frame False {
      n98 = for {
        tunnel: w410 -> [w412] mode=indexing
        tunnel: [w411] -> w409 mode=indexing
        n99 = Unbundle By Name(w412) -> ("Custom Curve Name"=w411:string)
      }
    }
    frame True {
      n100 = for {
        tunnel: w415 -> [w417] mode=indexing
        tunnel: [w421] -> w414 mode=indexing
        tunnel: w413 -> [w419]
        n101 = Unbundle By Name(w417) -> ("Custom Curve Name"=w416:string)
        n102 = Concatenate Strings(w416, " [" ("RecordDelay"), w419, "]" ("string")) -> (w421:string)
      }
    }
  }
  n103 = case shown="True" w117 {
    tunnel: w54 -> [w423 w428]
    tunnel: [w422 w427] -> w33
    tunnel: w28 -> [_ w426]
    frame False {
      n104 = for {
        tunnel: w423 -> [w425] mode=indexing
        tunnel: [w424] -> w422 mode=indexing
        n105 = Unbundle By Name(w425) -> ("Custom Curve Name"=w424:string)
      }
    }
    frame True {
      n106 = for {
        tunnel: w428 -> [w430] mode=indexing
        tunnel: [w434] -> w427 mode=indexing
        tunnel: w426 -> [w432]
        n107 = Unbundle By Name(w430) -> ("Custom Curve Name"=w429:string)
        n108 = Concatenate Strings(w429, " [" ("RecordDelay"), w432, "]" ("string")) -> (w434:string)
      }
    }
  }
  n109 = case shown="False" w117 {
    tunnel: w66 -> [w436 w441]
    tunnel: [w435 w439] -> w32
    tunnel: w28 -> [_ w440]
    frame False {
      n110 = for {
        tunnel: w436 -> [w438] mode=indexing
        tunnel: [w437] -> w435 mode=indexing
        n111 = Unbundle By Name(w438) -> ("Custom Curve Name"=w437:string)
      }
    }
    frame True {
      n112 = for {
        tunnel: w441 -> [w443] mode=indexing
        tunnel: w440 -> [w445]
        tunnel: [w444] -> w439 mode=indexing
        n113 = Unbundle By Name(w443) -> ("Custom Curve Name"=w442:string)
        n114 = Concatenate Strings(w442, " [" ("RecordDelay"), w445, "]" ("string")) -> (w444:string)
      }
    }
  }
  n115 = Index Array(array="Curve array") -> (element=w118:T5)  [unwired: 1 in]
  n116 = for {
    tunnel: w37 -> [w464]
    shift-right: [w462] -> w43
    shift-left: "Wave out" -> [w463]
    tunnel: w32 -> [w459] mode=indexing
    tunnel: w63 -> [w455] mode=indexing
    tunnel: w62 -> [w458] mode=indexing
    tunnel: ["Wave" ("string")] -> w23 mode=indexing
    n117 = Unbundle By Name(w458) -> ("display X"=w457:bool, "display Y"=w456:bool)
    n118 = Unbundle By Name(w455) -> ("X unit"=w454:string, "X data"=w453:u16, "Y unit"=w452:string, "Y data Time"=w451:u16, "X dB ref"=w450:dbl)
    n119 = Index Array(array=w463) -> (element=w461:T3)  [unwired: 1 in]
    n120 = Bundle By Name(cluster=w461, "Step No."=w464, "Name"=w459, "X unit"=w454, "X data"=w453, "Y unit"=w452, "Y data"=w451, "Y axis"=u16 1, "Y dB ref"=w450, "display X"=w457, "display Y"=w456) -> (w460:T3)
    n121 = Insert Into Array(array=w463, new element=w460) -> (w462:T3[])  [unwired: 1 in]
  }
  n122 = for {
    tunnel: w118 -> [w484]
    tunnel: w37 -> [w483]
    shift-right: [w481] -> w45
    shift-left: "Curve array" -> [w482]
    tunnel: w34 -> [w478] mode=indexing
    tunnel: w9 -> [w477] mode=indexing
    tunnel: w8 -> [w469] mode=indexing
    tunnel: ["Curve" ("string")] -> w25 mode=indexing
    n123 = Unbundle By Name(w477) -> ("X unit"=w476:string, "X data"=w475:u16, "Y unit"=w474:string, "Y data Time"=w473:u16, "X axis"=w472:u16, "X dB ref"=w471:dbl, "Y dB ref"=w470:dbl)  [unwired: 1 out]
    n124 = Unbundle By Name(w469) -> ("display X"=w468:bool, "display Y"=w467:bool, "display Z"=w466:bool)
    n125 = Bundle By Name(cluster=w484, "Name"=w478, "single val"=FALSE, "Step No."=w483, "X data"=w475, "Y data"=w473, "X axis"=w472, "X unit"=w476, "Y unit"=w474, "X dB ref"=w471, "Y dB ref"=w470, "display X"=w468, "display Y"=w467, "display Z"=w466) -> (w480:T5)
    n126 = Insert Into Array(array=w482, new element=w480) -> (w481:T4)  [unwired: 1 in]
  }
  n127 = for {
    tunnel: w33 -> [w500] mode=indexing
    tunnel: w118 -> [w501]
    tunnel: w37 -> [w499]
    shift-right: [w497] -> w44
    shift-left: "Curve array" -> [w498]
    tunnel: w113 -> [w493] mode=indexing
    tunnel: w112 -> [w486] mode=indexing
    tunnel: ["Value" ("string")] -> w24 mode=indexing
    w495 = u16 1 ("X data")
    n128 = Unbundle By Name(w493) -> ("display X"=w492:bool, "display Y"=w491:bool, "display Z"=w490:bool)
    n129 = Unbundle By Name(w486) -> ("X unit"=w489:string, "Y unit"=w488:string, "Y unit"=w487:string)  [unwired: 3 out]
    n130 = Bundle By Name(cluster=w501, "Name"=w500, "single val"=TRUE, "Step No."=w499, "X data"=w495, "Y data"=w495, "Z data"=w495, "X axis"=w495, "Y axis"=w495, "Z axis"=w495, "X unit"=w489, "Y unit"=w488, "Z unit"=w487, "display X"=w492, "display Y"=w491, "display Z"=w490) -> (w496:T5)
    n131 = Insert Into Array(array=w498, new element=w496) -> (w497:T4)  [unwired: 1 in]
  }
  n132 = Build Array (concatenate)(w25, w24, w23) -> (→"New Custom Type( Channel case)":string[])
  n133 = Build Array (concatenate)(w34, w33, w32) -> (→"New Custom Name( Channel case)":string[])
  n134 = case shown="False" w38 {
    tunnel: "TOTAL_CURVES" ("Type In") -> [w509 _]
    tunnel: w45 -> [w508 w512]
    tunnel: w44 -> [w507 w511]
    tunnel: w43 -> [w506 w510]
    tunnel: [w505 w512] -> w42
    tunnel: [w504 w511] -> w41
    tunnel: [w503 w510] -> w40
    tunnel: w39 -> [w502 _]
    frame False {
      n135 = call "CRYPrefix Curve Name.vi"("Type In"=w509, "Curves In"=w508, "Values In"=w507, "Waves In"=w506, "Repeat State Array In"=w502) -> ("Curves Out"=w505:T4, "Values Out"=w504:T4, "Waves Out"=w503:T20)  [unwired: 7 in, 1 out]
    }
    frame True {
    }
  }
  n136 = Concatenate Strings(" [" ("RecordDelay"), w28, "]" ("string")) -> (→"Signal Type":string)
  n137 = case shown="True" "InsertSocket?" {
    tunnel: [_ w519] -> w122
    tunnel: "Type In" -> [_ w518]
    tunnel: w49 -> [_ w517]
    tunnel: w42 -> [_ w516]
    tunnel: w41 -> [_ w515]
    tunnel: w40 -> [_ w514]
    tunnel: w37 -> [_ w513]
    frame False {
    }
    frame True {
      n138 = call "CRYInsert Socket.vi"("sOption2"=w517, "Step No."=w513, "sOption1"=w518, "Waves"=w514, "Values"=w515, "Curves"=w516) -> ("Inserted Names Out"=w519:string[])  [unwired: 5 in]
    }
  }
  "Inserted Names Out" <- w122
